vi "Highlight Item in Tree.vi"(8 "error in":errorcluster, 10 "Tag":string, 11 "TreeControl in":refnum<vi>) -> (0 "error out":errorcluster)   [LabVIEW 2020, in "Panther Dashboard.lvlib"]
uses:
  Panther Dashboard.lvlib
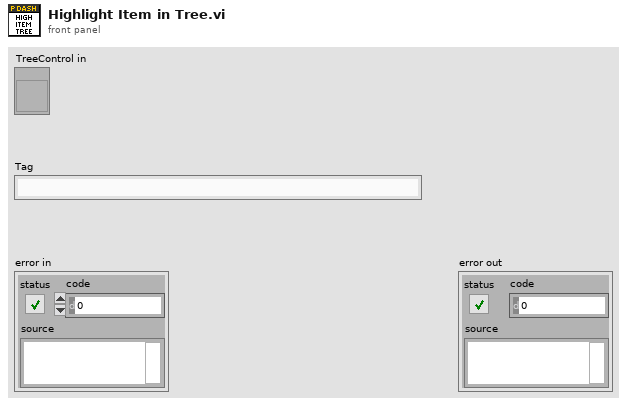
[diagram p1: front panel]
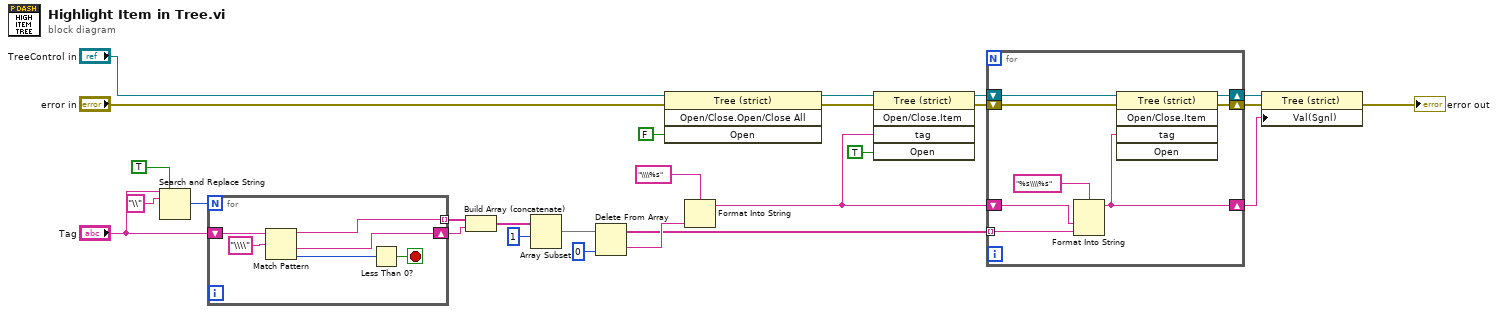
[diagram p0: block diagram]
diagram:
  n1 = Search and Replace String(replace all?=TRUE ("replace all? (F)"), input string="Tag", search string="\\") -> (number of replacements=w19:i32)  [unwired: 5 in, 3 out]
  n2 = for {
    N: w19 -> [_]
    tunnel: [w27] -> w18 mode=indexing
    shift-right: [w28] -> w17
    shift-left: "Tag" -> [w32]
    stop <- w29 stop-if-true
    n3 = Match Pattern(string=w32, regular expression="\\\\" ("search string")) -> (before substring=w27:string, after substring=w28:string, offset past match=w30:i32)  [unwired: 1 in, 1 out]
    n4 = Less Than 0?(x=w30) -> (x < 0?=w29:bool)
  }
  n5 = Build Array (concatenate)(w18, w17) -> (w16:string[])
  n6 = Array Subset(array=w16, index=1) -> (w13:string[])  [unwired: 1 in]
  n7 = Delete From Array(array=w13, index=0) -> (deleted portion=w12:string, array with subset deleted=w10:string[])  [unwired: 1 in]
  n8 = invoke class="Tree (strict)" method="Open/Close.Open/Close All"(reference="TreeControl in", error in="error in", "Open"=FALSE ("Open?")) -> (reference out=w7:refnum<vi>, error out=w24:errorcluster)  [unwired: 1 in, 2 out]
  n9 = Format Into String(format string="\\\\%s", w12) -> (resulting string=w5:string)  [unwired: 2 in, 1 out]
  n10 = invoke class="Tree (strict)" method="Open/Close.Item"(reference=w7, error in=w24, "tag"=w5, "Open"=TRUE ("Open?")) -> (reference out=w6:refnum<vi>, error out=w23:errorcluster)  [unwired: 1 in, 3 out]
  n11 = for {
    tunnel: w10 -> [w35] mode=indexing
    shift-right: [w33] -> w2
    shift-left: w5 -> [w36]
    shift-right: [w39] -> w25
    shift-left: w23 -> [w40]
    shift-right: [w37] -> w3
    shift-left: w6 -> [w38]
    n12 = Format Into String(format string="%s\\\\%s", w36, w35) -> (resulting string=w33:string)  [unwired: 2 in, 1 out]
    n13 = invoke class="Tree (strict)" method="Open/Close.Item"(reference=w38, error in=w40, "tag"=w33) -> (reference out=w37:refnum<vi>, error out=w39:errorcluster)  [unwired: 2 in, 3 out]
  }
  n14 = property class="Tree (strict)"(reference=w3, error in=w25, "Val(Sgnl)"=w2) -> (error out=→"error out":errorcluster)  [unwired: 1 out]
